vi "read_params.vi"(8 "error in (no error)":errorcluster, 11 "FeatureAgglomeration in":refnum<class "FeatureAgglomeration.lvclass">) -> (0 "error out":errorcluster, 2 "params":T1={"n_clusters"=2.0, "affinity"="euclidean", "memory"="None", "connectivity"={"connectivity_type"="None", "connectivity_list"=[]}, "compute_full_tree"={"compute_full_tree_type"="auto", "compute_full_tree_bool"=FALSE}, "linkage"="ward", "distance_threshold"={"distance_threshold_type"="None", "distance_threshold_float"=0.0}, "compute_distances"=FALSE}, 3 "FeatureAgglomeration out":refnum<class "FeatureAgglomeration.lvclass">)   [LabVIEW 2020, in "FeatureAgglomeration.lvclass"]
uses:
  FeatureAgglomeration.lvclass
  Controls/feature_agglomeration_params.ctl
  FeatureAgglomeration.lvclass/FeatureAgglomeration.ctl
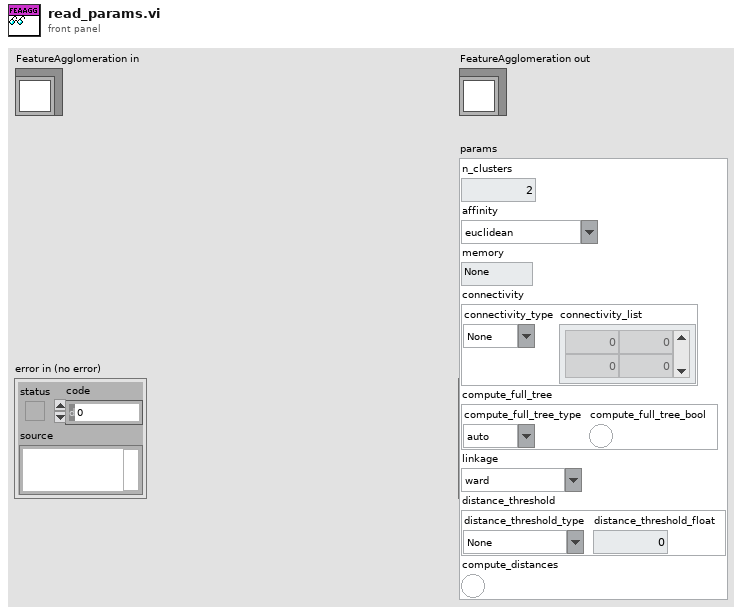
[diagram p1: front panel]
types:
  T1 = typedef "feature_agglomeration_params.ctl" = cluster{"n_clusters":dbl, "affinity":string, "memory":string, "connectivity":cluster{"connectivity_type":string, "connectivity_list":dbl[][]}, "compute_full_tree":cluster{"compute_full_tree_type":string, "compute_full_tree_bool":bool}, "linkage":string, "distance_threshold":cluster{"distance_threshold_type":string, "distance_threshold_float":dbl}, "compute_distances":bool}
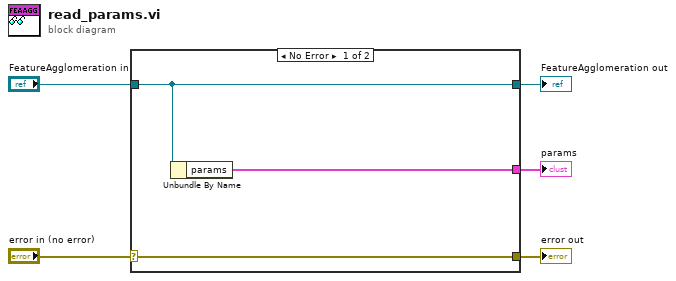
[diagram p0: block diagram]
diagram:
  n1 = case shown="No Error" "error in (no error)" {
    selector: "error in (no error)" -> [w8 w9]
    tunnel: [w8 w9] -> w4
    tunnel: [w7 w10] -> w2
    tunnel: "FeatureAgglomeration in" -> [w7 w10]
    tunnel: [w6 _] -> w1
    frame No Error {
      n2 = Unbundle By Name(w7) -> ("params"=w6:T1)
    }
    frame Error {
    }
  }
  "error out" <- w4
  "FeatureAgglomeration out" <- w2
  "params" <- w1
